vi "输入数据解析.vi"(0 "单个参数补充":dbl, 1 "从板号":dbl=1.0, 2 "主板二维码":string="BNET01", 3 "从板二维码":string="BNET01", 5 "主板引用":refnum<vi>, 7 "从板引用":refnum<vi>, 9 "主板选项":string="三级故障阀值", 11 "枚举":enum16{"主板", "从板"}(ring), 12 "快换":bool caption="快换写入") -> (4 "输出数组":dbl[][](array[numeric]), 6 "数组长度":dbl[](array[numeric]), 8 "循环次数":i32, 10 "命令":u32, 14 "名称":string[](array[string]), 15 "命令序号":u32[](array[numeric]))   [LabVIEW 2013] (continued)
          n4752 = Build Array(w12196) -> (w12195:dbl[][])
          n4753 = Build Array("二级故障阀值") -> (w12186:string[])
        }
        frame "SOC过低(3)" {
          n4754 = Unbundle By Name(w12405) -> ("一级故障 3"=w12406:refnum<vi>)
          n4755 = property class="Clust (严格)"(reference=w12406) -> ("Value"=w12404:T4)  [unwired: 1 in, 2 out]
          n4756 = for {
            N: 17 -> [_]
            tunnel: w12404 -> [w12416]
            shift-right: [w12413] -> w12410
            shift-left: dbl[] [] -> [w12414]
            i -> [w12417]
            n4757 = case shown="12" w12417 {
              tunnel: w12416 -> [w12418 w12429 w12440 w12450 w12460 w12470 w12482 w12494 w12506 w12518 w12530 w12542 w12554 w12566 w12573 w12582 w12591]
              tunnel: [w12419 w12430 w12441 w12451 w12461 w12472 w12484 w12496 w12508 w12520 w12532 w12543 w12556 w12568 w12572 w12581 w12593] -> w12415
              frame 0, Default {
                # "总电压过高"
                n4758 = disable-structure shown="启用" {
                  disable-tunnel: [w12425 w12428] -> w12421
                  disable-tunnel: [w12424 w12428] -> w12420
                  disable-tunnel: w12418 -> [w12423 _]
                  frame Disabled {
                    n4759 = Unbundle By Name(w12423) -> ("总电压过高"=w12422:dbl)
                    n4760 = call "输入分辨率计算-EV05.vi"("1字节?"=FALSE, "数值"=w12422, "分辨率"=0.1) -> ("低字节"=w12425:dbl, "高字节1"=w12424:dbl)  [unwired: 2 in, 5 out]
                  }
                  frame Enabled {
                    w12428 = 255 ("高字节1")
                  }
                }
                n4761 = Build Array(w12420, w12421) -> (w12419:i32[])
              }
              frame 1 {
                # "总电压过低"
                n4762 = disable-structure shown="启用" {
                  disable-tunnel: [w12436 w12439] -> w12432
                  disable-tunnel: [w12435 w12439] -> w12431
                  disable-tunnel: w12429 -> [w12434 _]
                  frame Disabled {
                    n4763 = Unbundle By Name(w12434) -> ("总电压过低"=w12433:dbl)
                    n4764 = call "输入分辨率计算-EV05.vi"("1字节?"=FALSE, "数值"=w12433, "分辨率"=0.1) -> ("低字节"=w12436:dbl, "高字节1"=w12435:dbl)  [unwired: 2 in, 5 out]
                  }
                  frame Enabled {
                    w12439 = 255 ("高字节1")
                  }
                }
                n4765 = Build Array(w12431, w12432) -> (w12430:i32[])
              }
              frame 2 {
                # "温度过高"
                n4766 = disable-structure shown="启用" {
                  disable-tunnel: [w12446 255 ("高字节1")] -> w12442
                  disable-tunnel: w12440 -> [w12444 _]
                  frame Disabled {
                    n4767 = Unbundle By Name(w12444) -> ("温度过高"=w12443:dbl)
                    n4768 = call "输入分辨率计算-EV05.vi"("1字节?"=TRUE, "数值"=w12443, "偏移量"=-40.0, "分辨率"=1.0) -> ("高字节1"=w12446:dbl)  [unwired: 1 in, 6 out]
                  }
                  frame Enabled {
                  }
                }
                n4769 = Build Array(w12442) -> (w12441:i32[])
              }
              frame 3 {
                # "温度过低"
                n4770 = disable-structure shown="启用" {
                  disable-tunnel: [w12456 255 ("高字节1")] -> w12452
                  disable-tunnel: w12450 -> [w12454 _]
                  frame Disabled {
                    n4771 = Unbundle By Name(w12454) -> ("温度过低"=w12453:dbl)
                    n4772 = call "输入分辨率计算-EV05.vi"("1字节?"=TRUE, "数值"=w12453, "偏移量"=-40.0, "分辨率"=1.0) -> ("高字节1"=w12456:dbl)  [unwired: 1 in, 6 out]
                  }
                  frame Enabled {
                  }
                }
                n4773 = Build Array(w12452) -> (w12451:i32[])
              }
              frame 4 {
                # "整组温度不均衡"
                n4774 = disable-structure shown="启用" {
                  disable-tunnel: [w12466 255 ("高字节1")] -> w12462
                  disable-tunnel: w12460 -> [w12464 _]
                  frame Disabled {
                    n4775 = Unbundle By Name(w12464) -> ("整组温度不均衡"=w12463:dbl)
                    n4776 = call "输入分辨率计算-EV05.vi"("1字节?"=TRUE, "数值"=w12463, "偏移量"=0.0, "分辨率"=1.0) -> ("高字节1"=w12466:dbl)  [unwired: 1 in, 6 out]
                  }
                  frame Enabled {
                  }
                }
                n4777 = Build Array(w12462) -> (w12461:i32[])
              }
              frame 5 {
                # "单组电压不均衡"
                n4778 = disable-structure shown="启用" {
                  disable-tunnel: [w12478 w12481] -> w12473
                  disable-tunnel: [w12476 w12481] -> w12471
                  disable-tunnel: w12470 -> [w12475 _]
                  frame Disabled {
                    n4779 = Unbundle By Name(w12475) -> ("单组电压不均衡"=w12474:dbl)
                    n4780 = call "输入分辨率计算-EV05.vi"("1字节?"=FALSE, "数值"=w12474, "偏移量"=0.0, "分辨率"=0.001) -> ("低字节"=w12476:dbl, "高字节1"=w12478:dbl)  [unwired: 1 in, 5 out]
                  }
                  frame Enabled {
                    w12481 = 255 ("高字节1")
                  }
                }
                n4781 = Build Array(w12473, w12471) -> (w12472:i32[])
              }
              frame 6 {
                # "整组电压不均衡"
                n4782 = disable-structure shown="启用" {
                  disable-tunnel: [w12490 w12493] -> w12485
                  disable-tunnel: [w12488 w12493] -> w12483
                  disable-tunnel: w12482 -> [w12487 _]
                  frame Disabled {
                    n4783 = Unbundle By Name(w12487) -> ("整组电压不均衡"=w12486:dbl)
                    n4784 = call "输入分辨率计算-EV05.vi"("1字节?"=FALSE, "数值"=w12486, "偏移量"=0.0, "分辨率"=0.001) -> ("低字节"=w12488:dbl, "高字节1"=w12490:dbl)  [unwired: 1 in, 5 out]
                  }
                  frame Enabled {
                    w12493 = 255 ("高字节1")
                  }
                }
                n4785 = Build Array(w12485, w12483) -> (w12484:i32[])
              }
              frame 7 {
                # "单体电压过高"
                n4786 = disable-structure shown="启用" {
                  disable-tunnel: [w12502 w12505] -> w12497
                  disable-tunnel: [w12500 w12505] -> w12495
                  disable-tunnel: w12494 -> [w12499 _]
                  frame Disabled {
                    n4787 = Unbundle By Name(w12499) -> ("单体电压过高"=w12498:dbl)
                    n4788 = call "输入分辨率计算-EV05.vi"("1字节?"=FALSE, "数值"=w12498, "偏移量"=0.0, "分辨率"=0.001) -> ("低字节"=w12500:dbl, "高字节1"=w12502:dbl)  [unwired: 1 in, 5 out]
                  }
                  frame Enabled {
                    w12505 = 255 ("高字节1")
                  }
                }
                n4789 = Build Array(w12497, w12495) -> (w12496:i32[])
              }
              frame 8 {
                # "单体电压过低"
                n4790 = disable-structure shown="启用" {
                  disable-tunnel: [w12514 w12517] -> w12509
                  disable-tunnel: [w12512 w12517] -> w12507
                  disable-tunnel: w12506 -> [w12511 _]
                  frame Disabled {
                    n4791 = Unbundle By Name(w12511) -> ("单体电压过低"=w12510:dbl)
                    n4792 = call "输入分辨率计算-EV05.vi"("1字节?"=FALSE, "数值"=w12510, "偏移量"=0.0, "分辨率"=0.001) -> ("低字节"=w12512:dbl, "高字节1"=w12514:dbl)  [unwired: 1 in, 5 out]
                  }
                  frame Enabled {
                    w12517 = 255 ("高字节1")
                  }
                }
                n4793 = Build Array(w12509, w12507) -> (w12508:i32[])
              }
              frame 9 {
                # "充电电流过高"
                n4794 = disable-structure shown="启用" {
                  disable-tunnel: [w12526 w12529] -> w12521
                  disable-tunnel: [w12524 w12529] -> w12519
                  disable-tunnel: w12518 -> [w12523 _]
                  frame Disabled {
                    n4795 = Unbundle By Name(w12523) -> ("充电电流过高"=w12522:dbl)
                    n4796 = call "输入分辨率计算-EV05.vi"("1字节?"=FALSE, "数值"=w12522, "偏移量"=-3000.0, "分辨率"=0.1) -> ("低字节"=w12524:dbl, "高字节1"=w12526:dbl)  [unwired: 1 in, 5 out]
                  }
                  frame Enabled {
                    w12529 = 255 ("高字节1")
                  }
                }
                n4797 = Build Array(w12521, w12519) -> (w12520:i32[])
              }
              frame 10 {
                # "放电电流过高"
                n4798 = disable-structure shown="启用" {
                  disable-tunnel: [w12538 w12541] -> w12533
                  disable-tunnel: [w12536 w12541] -> w12531
                  disable-tunnel: w12530 -> [w12535 _]
                  frame Disabled {
                    n4799 = Unbundle By Name(w12535) -> ("放电电流过高"=w12534:dbl)
                    n4800 = call "输入分辨率计算-EV05.vi"("1字节?"=FALSE, "数值"=w12534, "偏移量"=-3000.0, "分辨率"=0.1) -> ("低字节"=w12536:dbl, "高字节1"=w12538:dbl)  [unwired: 1 in, 5 out]
                  }
                  frame Enabled {
                    w12541 = 255 ("高字节1")
                  }
                }
                n4801 = Build Array(w12533, w12531) -> (w12532:i32[])
              }
              frame 11 {
                # "单组温度不均衡"
                n4802 = disable-structure shown="启用" {
                  disable-tunnel: [w12548 255 ("高字节1")] -> w12544
                  disable-tunnel: w12542 -> [w12546 _]
                  frame Disabled {
                    n4803 = Unbundle By Name(w12546) -> ("单组温度不均衡"=w12545:dbl)
                    n4804 = call "输入分辨率计算-EV05.vi"("1字节?"=TRUE, "数值"=w12545, "偏移量"=0.0, "分辨率"=1.0) -> ("高字节1"=w12548:dbl)  [unwired: 1 in, 6 out]
                  }
                  frame Enabled {
                  }
                }
                n4805 = Build Array(w12544) -> (w12543:i32[])
              }
              frame 12 {
                # "SOC过高"
                n4806 = Unbundle By Name(w12554) -> ("SOC过高"=w12553:dbl)
                n4807 = call "输入分辨率计算-EV05.vi"("1字节?"=FALSE, "数值"=w12553, "偏移量"=0.0, "分辨率"=0.1) -> ()  [unwired: 1 in, 7 out]
                n4808 = disable-structure shown="启用" {
                  disable-tunnel: _ -> [w12560 _]
                  disable-tunnel: [w12560 255 ("高字节1")] -> w12552
                  disable-tunnel: [w12559 i32[] [] ("低位子数组")] -> _
                  disable-tunnel: _ -> [w12559 _]
                  frame Disabled {
                  }
                  frame Enabled {
                  }
                }
                n4809 = Build Array(w12552, w12552) -> (w12556:i32[])
              }
              frame 13 {
                n4810 = Unbundle By Name(w12566) -> ("SOC过低"=w12565:dbl)
                n4811 = call "输入分辨率计算-EV05.vi"("1字节?"=FALSE, "数值"=w12565, "偏移量"=0.0, "分辨率"=0.1) -> ("低字节"=w12563:dbl, "高字节1"=w12564:dbl)  [unwired: 1 in, 5 out]
                n4812 = Build Array(w12564, w12563) -> (w12568:dbl[])
              }
              frame 14 {
                # "内阻过大"
                n4813 = disable-structure shown="启用" {
                  disable-tunnel: w12573 -> [w12578 _]
                  disable-tunnel: [w12574 255 ("高字节1")] -> w12571
                  frame Disabled {
                    n4814 = Unbundle By Name(w12578) -> ("内阻过大"=w12577:dbl)
                    n4815 = call "输入分辨率计算-EV05.vi"("1字节?"=TRUE, "数值"=w12577, "分辨率"=0.1) -> ("高字节1"=w12574:dbl)  [unwired: 2 in, 6 out]
                  }
                  frame Enabled {
                  }
                }
                n4816 = Build Array(w12571) -> (w12572:i32[])
              }
              frame 15 {
                # "极柱温度过高"
                n4817 = disable-structure shown="启用" {
                  disable-tunnel: w12582 -> [w12588 _]
                  disable-tunnel: [w12584 255 ("高字节1")] -> w12580
                  frame Disabled {
                    n4818 = Unbundle By Name(w12588) -> ("极柱温度过高"=w12587:dbl)
                    n4819 = call "输入分辨率计算-EV05.vi"("1字节?"=TRUE, "数值"=w12587, "偏移量"=-40.0, "分辨率"=1.0) -> ("高字节1"=w12584:dbl)  [unwired: 1 in, 6 out]
                  }
                  frame Enabled {
                  }
                }
                n4820 = Build Array(w12580) -> (w12581:i32[])
              }
              frame 16 {
                # "SOH过低"
                n4821 = disable-structure shown="启用" {
                  disable-tunnel: [w12605 w12613] -> w12592
                  disable-tunnel: w12591 -> [w12602 _]
                  disable-tunnel: [w12594 w12613] -> w12590
                  frame Disabled {
                    n4822 = Unbundle By Name(w12602) -> ("SOH过低"=w12601:dbl)
                    n4823 = call "输入分辨率计算-EV05.vi"("1字节?"=FALSE, "数值"=w12601, "偏移量"=0.0, "分辨率"=0.1) -> ("低字节"=w12603:dbl, "高字节1"=w12604:dbl)  [unwired: 1 in, 5 out]
                    n4824 = call "二进制解析-8.6.vi"("索引"=4, "数值"=w12604) -> ("低位子数组"=w12607:i32[])  [unwired: 3 out]
                    n4825 = call "二进制解析-8.6.vi"("索引"=4, "数值"=w12603) -> ("低位子数组"=w12596:i32[], "高位子数组"=w12606:i32[])  [unwired: 2 out]
                    n4826 = call "二进制解析-8.6.vi"("索引"=4, "数值"=0) -> ("低位子数组"=w12597:i32[])  [unwired: 3 out]
                    n4827 = Insert Into Array(array=w12607, new element=w12606) -> (w12600:i32[])  [unwired: 1 in]
                    n4828 = Insert Into Array(array=w12596, new element=w12597) -> (w12595:i32[])  [unwired: 1 in]
                    n4829 = call "数值二进制转十进制-8.6.vi"("子数组"=w12600) -> ("十进制数值"=w12605:i32)  [unwired: 4 out]
                    n4830 = call "数值二进制转十进制-8.6.vi"("子数组"=w12595) -> ("十进制数值"=w12594:i32)  [unwired: 4 out]
                  }
                  frame Enabled {
                    w12613 = 255 ("高字节1")
                  }
                }
                n4831 = Build Array(w12592, w12590) -> (w12593:i32[])
              }
            }
            n4832 = Insert Into Array(array=w12414, new element=w12415) -> (w12413:dbl[])  [unwired: 1 in]
          }
          n4833 = Build Array(w12410) -> (w12409:dbl[][])
          n4834 = Build Array("三级故障阀值") -> (w12400:string[])
        }
        frame "二级故障阀值" {
          n4835 = Unbundle By Name(w12619) -> ("一级故障 2"=w12620:refnum<vi>)
          n4836 = property class="Clust (严格)"(reference=w12620) -> ("Value"=w12618:T4)  [unwired: 1 in, 2 out]
          n4837 = for {
            N: 17 -> [_]
            tunnel: w12618 -> [w12630]
            shift-right: [w12627] -> w12624
            shift-left: dbl[] [] -> [w12628]
            i -> [w12631]
            n4838 = case shown="4" w12631 {
              tunnel: w12630 -> [w12633 w12640 w12647 w12654 w12661 w12667 w12675 w12683 w12691 w12699 w12707 w12715 w12723 w12731 w12741 w12748 w12752]
              tunnel: [w12634 w12641 w12649 w12656 w12662 w12670 w12678 w12686 w12694 w12702 w12710 w12716 w12725 w12733 w12740 w12747 w12754] -> w12629
              frame 0, Default {
                # "总电压过高"
                n4839 = Unbundle By Name(w12633) -> ("总电压过高"=w12632:dbl)
                n4840 = call "输入分辨率计算-EV05.vi"("1字节?"=FALSE, "数值"=w12632, "分辨率"=0.1) -> ("低字节"=w12636:dbl, "高字节1"=w12635:dbl)  [unwired: 2 in, 5 out]
                n4841 = Build Array(w12635, w12636) -> (w12634:dbl[])
              }
              frame 1 {
                # "总电压过低"
                n4842 = Unbundle By Name(w12640) -> ("总电压过低"=w12639:dbl)
                n4843 = call "输入分辨率计算-EV05.vi"("1字节?"=FALSE, "数值"=w12639, "分辨率"=0.1) -> ("低字节"=w12643:dbl, "高字节1"=w12642:dbl)  [unwired: 2 in, 5 out]
                n4844 = Build Array(w12642, w12643) -> (w12641:dbl[])
              }
              frame 2 {
                # "温度过高"
                n4845 = Unbundle By Name(w12647) -> ("温度过高"=w12646:dbl)
                n4846 = call "输入分辨率计算-EV05.vi"("1字节?"=TRUE, "数值"=w12646, "偏移量"=-40.0, "分辨率"=1.0) -> ("高字节1"=w12650:dbl)  [unwired: 1 in, 6 out]
                n4847 = Build Array(w12650) -> (w12649:dbl[])
              }
              frame 3 {
                # "温度过低"
                n4848 = Unbundle By Name(w12654) -> ("温度过低"=w12653:dbl)
                n4849 = call "输入分辨率计算-EV05.vi"("1字节?"=TRUE, "数值"=w12653, "偏移量"=-40.0, "分辨率"=1.0) -> ("高字节1"=w12657:dbl)  [unwired: 1 in, 6 out]
                n4850 = Build Array(w12657) -> (w12656:dbl[])
              }
              frame 4 {
                # "整组温度不均衡"
                n4851 = Unbundle By Name(w12661) -> ("整组温度不均衡"=w12660:dbl)
                n4852 = call "输入分辨率计算-EV05.vi"("1字节?"=TRUE, "数值"=w12660, "分辨率"=1.0) -> ("高字节1"=w12663:dbl)  [unwired: 2 in, 6 out]
                n4853 = Build Array(w12663) -> (w12662:dbl[])
              }
              frame 5 {
                # "单组电压不均衡"
                n4854 = Unbundle By Name(w12667) -> ("单组电压不均衡"=w12666:dbl)
                n4855 = call "输入分辨率计算-EV05.vi"("1字节?"=FALSE, "数值"=w12666, "偏移量"=0.0, "分辨率"=0.001) -> ("低字节"=w12668:dbl, "高字节1"=w12671:dbl)  [unwired: 1 in, 5 out]
                n4856 = Build Array(w12671, w12668) -> (w12670:dbl[])
              }
              frame 6 {
                # "整组电压不均衡"
                n4857 = Unbundle By Name(w12675) -> ("整组电压不均衡"=w12674:dbl)
                n4858 = call "输入分辨率计算-EV05.vi"("1字节?"=FALSE, "数值"=w12674, "偏移量"=0.0, "分辨率"=0.001) -> ("低字节"=w12676:dbl, "高字节1"=w12679:dbl)  [unwired: 1 in, 5 out]
                n4859 = Build Array(w12679, w12676) -> (w12678:dbl[])
              }
              frame 7 {
                # "单体电压过高"
                n4860 = Unbundle By Name(w12683) -> ("单体电压过高"=w12682:dbl)
                n4861 = call "输入分辨率计算-EV05.vi"("1字节?"=FALSE, "数值"=w12682, "偏移量"=0.0, "分辨率"=0.001) -> ("低字节"=w12684:dbl, "高字节1"=w12687:dbl)  [unwired: 1 in, 5 out]
                n4862 = Build Array(w12687, w12684) -> (w12686:dbl[])
              }
              frame 8 {
                # "单体电压过低"
                n4863 = Unbundle By Name(w12691) -> ("单体电压过低"=w12690:dbl)
                n4864 = call "输入分辨率计算-EV05.vi"("1字节?"=FALSE, "数值"=w12690, "偏移量"=0.0, "分辨率"=0.001) -> ("低字节"=w12692:dbl, "高字节1"=w12695:dbl)  [unwired: 1 in, 5 out]
                n4865 = Build Array(w12695, w12692) -> (w12694:dbl[])
              }
              frame 9 {
                # "充电电流过高"
                n4866 = Unbundle By Name(w12699) -> ("充电电流过高"=w12698:dbl)
                n4867 = call "输入分辨率计算-EV05.vi"("1字节?"=FALSE, "数值"=w12698, "偏移量"=0.0, "分辨率"=0.1) -> ("低字节"=w12700:dbl, "高字节1"=w12703:dbl)  [unwired: 1 in, 5 out]
                n4868 = Build Array(w12703, w12700) -> (w12702:dbl[])
              }
              frame 10 {
                # "放电电流过高"
                n4869 = Unbundle By Name(w12707) -> ("放电电流过高"=w12706:dbl)
                n4870 = call "输入分辨率计算-EV05.vi"("1字节?"=FALSE, "数值"=w12706, "偏移量"=0.0, "分辨率"=0.1) -> ("低字节"=w12708:dbl, "高字节1"=w12711:dbl)  [unwired: 1 in, 5 out]
                n4871 = Build Array(w12711, w12708) -> (w12710:dbl[])
              }
              frame 11 {
                # "单组温度不均衡"
                n4872 = Unbundle By Name(w12715) -> ("单组温度不均衡"=w12714:dbl)
                n4873 = call "输入分辨率计算-EV05.vi"("1字节?"=TRUE, "数值"=w12714, "分辨率"=1.0) -> ("高字节1"=w12717:dbl)  [unwired: 2 in, 6 out]
                n4874 = Build Array(w12717) -> (w12716:dbl[])
              }
              frame 12 {
                # "SOC过高"
                n4875 = Unbundle By Name(w12723) -> ("SOC过高"=w12722:dbl)
                n4876 = call "输入分辨率计算-EV05.vi"("1字节?"=FALSE, "数值"=w12722, "偏移量"=0.0, "分辨率"=0.1) -> ("低字节"=w12720:dbl, "高字节1"=w12721:dbl)  [unwired: 1 in, 5 out]
                n4877 = Build Array(w12721, w12720) -> (w12725:dbl[])
              }
              frame 13 {
                # "SOC过低"
                n4878 = Unbundle By Name(w12731) -> ("SOC过低"=w12730:dbl)
                n4879 = call "输入分辨率计算-EV05.vi"("1字节?"=FALSE, "数值"=w12730, "偏移量"=0.0, "分辨率"=0.1) -> ("低字节"=w12728:dbl, "高字节1"=w12729:dbl)  [unwired: 1 in, 5 out]
                n4880 = Build Array(w12729, w12728) -> (w12733:dbl[])
              }
              frame 14 {
                # "内阻过大"
                n4881 = Unbundle By Name(w12741) -> ("内阻过大"=w12739:dbl)
                n4882 = call "输入分辨率计算-EV05.vi"("1字节?"=TRUE, "数值"=w12739, "分辨率"=0.1) -> ("高字节1"=w12736:dbl)  [unwired: 2 in, 6 out]
                n4883 = Build Array(w12736) -> (w12740:dbl[])
              }
              frame 15 {
                # "极柱温度过高"
                n4884 = Unbundle By Name(w12748) -> ("极柱温度过高"=w12746:dbl)
                n4885 = call "输入分辨率计算-EV05.vi"("1字节?"=TRUE, "数值"=w12746, "偏移量"=-40.0, "分辨率"=1.0) -> ("高字节1"=w12743:dbl)  [unwired: 1 in, 6 out]
                n4886 = Build Array(w12743) -> (w12747:dbl[])
              }
              frame 16 {
                # "SOH过低"
                n4887 = Unbundle By Name(w12752) -> ("SOH过低"=w12751:dbl)
                n4888 = call "输入分辨率计算-EV05.vi"("1字节?"=FALSE, "数值"=w12751, "偏移量"=0.0, "分辨率"=0.1) -> ("低字节"=w12749:dbl, "高字节1"=w12750:dbl)  [unwired: 1 in, 5 out]
                n4889 = Build Array(w12750, w12749) -> (w12754:dbl[])
              }
            }
            n4890 = Insert Into Array(array=w12628, new element=w12629) -> (w12627:dbl[])  [unwired: 1 in]
          }
          n4891 = Build Array(w12624) -> (w12623:dbl[][])
          n4892 = Build Array("二级故障阀值") -> (w12614:string[])
        }
        frame "三级故障阀值" {
          n4893 = Unbundle By Name(w12762) -> ("一级故障 3"=w12763:refnum<vi>)
          n4894 = property class="Clust (严格)"(reference=w12763) -> ("Value"=w12761:T4)  [unwired: 1 in, 2 out]
          n4895 = for {
            N: 17 -> [_]
            tunnel: w12761 -> [w12773]
            shift-right: [w12770] -> w12767
            shift-left: dbl[] [] -> [w12771]
            i -> [w12774]
            n4896 = case shown="11" w12774 {
              tunnel: w12773 -> [w12776 w12783 w12790 w12797 w12804 w12810 w12818 w12826 w12834 w12842 w12850 w12858 w12866 w12874 w12884 w12891 w12895]
              tunnel: [w12777 w12784 w12792 w12799 w12805 w12813 w12821 w12829 w12837 w12845 w12853 w12859 w12868 w12876 w12883 w12890 w12897] -> w12772
              frame 0, Default {
                # "总电压过高"
                n4897 = Unbundle By Name(w12776) -> ("总电压过高"=w12775:dbl)
                n4898 = call "输入分辨率计算-EV05.vi"("1字节?"=FALSE, "数值"=w12775, "分辨率"=0.1) -> ("低字节"=w12779:dbl, "高字节1"=w12778:dbl)  [unwired: 2 in, 5 out]
                n4899 = Build Array(w12778, w12779) -> (w12777:dbl[])
              }
              frame 1 {
                # "总电压过低"
                n4900 = Unbundle By Name(w12783) -> ("总电压过低"=w12782:dbl)
                n4901 = call "输入分辨率计算-EV05.vi"("1字节?"=FALSE, "数值"=w12782, "分辨率"=0.1) -> ("低字节"=w12786:dbl, "高字节1"=w12785:dbl)  [unwired: 2 in, 5 out]
                n4902 = Build Array(w12785, w12786) -> (w12784:dbl[])
              }
              frame 2 {
                # "温度过高"
                n4903 = Unbundle By Name(w12790) -> ("温度过高"=w12789:dbl)
                n4904 = call "输入分辨率计算-EV05.vi"("1字节?"=TRUE, "数值"=w12789, "偏移量"=-40.0, "分辨率"=1.0) -> ("高字节1"=w12793:dbl)  [unwired: 1 in, 6 out]
                n4905 = Build Array(w12793) -> (w12792:dbl[])
              }
              frame 3 {
                # "温度过低"
                n4906 = Unbundle By Name(w12797) -> ("温度过低"=w12796:dbl)
                n4907 = call "输入分辨率计算-EV05.vi"("1字节?"=TRUE, "数值"=w12796, "偏移量"=-40.0, "分辨率"=1.0) -> ("高字节1"=w12800:dbl)  [unwired: 1 in, 6 out]
                n4908 = Build Array(w12800) -> (w12799:dbl[])
              }
              frame 4 {
                # "整组温度不均衡"
                n4909 = Unbundle By Name(w12804) -> ("整组温度不均衡"=w12803:dbl)
                n4910 = call "输入分辨率计算-EV05.vi"("1字节?"=TRUE, "数值"=w12803, "分辨率"=1.0) -> ("高字节1"=w12806:dbl)  [unwired: 2 in, 6 out]
                n4911 = Build Array(w12806) -> (w12805:dbl[])
              }
              frame 5 {
                # "单组电压不均衡"
                n4912 = Unbundle By Name(w12810) -> ("单组电压不均衡"=w12809:dbl)
                n4913 = call "输入分辨率计算-EV05.vi"("1字节?"=FALSE, "数值"=w12809, "偏移量"=0.0, "分辨率"=0.001) -> ("低字节"=w12811:dbl, "高字节1"=w12814:dbl)  [unwired: 1 in, 5 out]
                n4914 = Build Array(w12814, w12811) -> (w12813:dbl[])
              }
              frame 6 {
                # "整组电压不均衡"
                n4915 = Unbundle By Name(w12818) -> ("整组电压不均衡"=w12817:dbl)
                n4916 = call "输入分辨率计算-EV05.vi"("1字节?"=FALSE, "数值"=w12817, "偏移量"=0.0, "分辨率"=0.001) -> ("低字节"=w12819:dbl, "高字节1"=w12822:dbl)  [unwired: 1 in, 5 out]
                n4917 = Build Array(w12822, w12819) -> (w12821:dbl[])
              }
              frame 7 {
                # "单体电压过高"
                n4918 = Unbundle By Name(w12826) -> ("单体电压过高"=w12825:dbl)
                n4919 = call "输入分辨率计算-EV05.vi"("1字节?"=FALSE, "数值"=w12825, "偏移量"=0.0, "分辨率"=0.001) -> ("低字节"=w12827:dbl, "高字节1"=w12830:dbl)  [unwired: 1 in, 5 out]
                n4920 = Build Array(w12830, w12827) -> (w12829:dbl[])
              }
              frame 8 {
                # "单体电压过低"
                n4921 = Unbundle By Name(w12834) -> ("单体电压过低"=w12833:dbl)
                n4922 = call "输入分辨率计算-EV05.vi"("1字节?"=FALSE, "数值"=w12833, "偏移量"=0.0, "分辨率"=0.001) -> ("低字节"=w12835:dbl, "高字节1"=w12838:dbl)  [unwired: 1 in, 5 out]
                n4923 = Build Array(w12838, w12835) -> (w12837:dbl[])
              }
              frame 9 {
                # "充电电流过高"
                n4924 = Unbundle By Name(w12842) -> ("充电电流过高"=w12841:dbl)
                n4925 = call "输入分辨率计算-EV05.vi"("1字节?"=FALSE, "数值"=w12841, "偏移量"=0.0, "分辨率"=0.1) -> ("低字节"=w12843:dbl, "高字节1"=w12846:dbl)  [unwired: 1 in, 5 out]
                n4926 = Build Array(w12846, w12843) -> (w12845:dbl[])
              }
              frame 10 {
                # "放电电流过高"
                n4927 = Unbundle By Name(w12850) -> ("放电电流过高"=w12849:dbl)
                n4928 = call "输入分辨率计算-EV05.vi"("1字节?"=FALSE, "数值"=w12849, "偏移量"=0.0, "分辨率"=0.1) -> ("低字节"=w12851:dbl, "高字节1"=w12854:dbl)  [unwired: 1 in, 5 out]
                n4929 = Build Array(w12854, w12851) -> (w12853:dbl[])
              }
              frame 11 {
                # "单组温度不均衡"
                n4930 = Unbundle By Name(w12858) -> ("单组温度不均衡"=w12857:dbl)
                n4931 = call "输入分辨率计算-EV05.vi"("1字节?"=TRUE, "数值"=w12857, "分辨率"=1.0) -> ("高字节1"=w12860:dbl)  [unwired: 2 in, 6 out]
                n4932 = Build Array(w12860) -> (w12859:dbl[])
              }
              frame 12 {
                # "SOC过高"
                n4933 = Unbundle By Name(w12866) -> ("SOC过高"=w12865:dbl)
                n4934 = call "输入分辨率计算-EV05.vi"("1字节?"=FALSE, "数值"=w12865, "偏移量"=0.0, "分辨率"=0.1) -> ("低字节"=w12863:dbl, "高字节1"=w12864:dbl)  [unwired: 1 in, 5 out]
                n4935 = Build Array(w12864, w12863) -> (w12868:dbl[])
              }
              frame 13 {
                # "SOC过低"
                n4936 = Unbundle By Name(w12874) -> ("SOC过低"=w12873:dbl)
                n4937 = call "输入分辨率计算-EV05.vi"("1字节?"=FALSE, "数值"=w12873, "偏移量"=0.0, "分辨率"=0.1) -> ("低字节"=w12871:dbl, "高字节1"=w12872:dbl)  [unwired: 1 in, 5 out]
                n4938 = Build Array(w12872, w12871) -> (w12876:dbl[])
              }
              frame 14 {
                # "内阻过大"
                n4939 = Unbundle By Name(w12884) -> ("内阻过大"=w12882:dbl)
                n4940 = call "输入分辨率计算-EV05.vi"("1字节?"=TRUE, "数值"=w12882, "分辨率"=0.1) -> ("高字节1"=w12879:dbl)  [unwired: 2 in, 6 out]
                n4941 = Build Array(w12879) -> (w12883:dbl[])
              }
              frame 15 {
                # "极柱温度过高"
                n4942 = Unbundle By Name(w12891) -> ("极柱温度过高"=w12889:dbl)
                n4943 = call "输入分辨率计算-EV05.vi"("1字节?"=TRUE, "数值"=w12889, "偏移量"=-40.0, "分辨率"=1.0) -> ("高字节1"=w12886:dbl)  [unwired: 1 in, 6 out]
                n4944 = Build Array(w12886) -> (w12890:dbl[])
              }
              frame 16 {
                # "SOH过低"
                n4945 = Unbundle By Name(w12895) -> ("SOH过低"=w12894:dbl)
                n4946 = call "输入分辨率计算-EV05.vi"("1字节?"=FALSE, "数值"=w12894, "偏移量"=0.0, "分辨率"=0.1) -> ("低字节"=w12892:dbl, "高字节1"=w12893:dbl)  [unwired: 1 in, 5 out]
                n4947 = Build Array(w12893, w12892) -> (w12897:dbl[])
              }
            }
            n4948 = Insert Into Array(array=w12771, new element=w12772) -> (w12770:dbl[])  [unwired: 1 in]
          }
          n4949 = Build Array(w12767) -> (w12766:dbl[][])
          n4950 = Build Array("三级故障阀值") -> (w12757:string[])
        }
        frame "加热控制参数" {
          n4951 = Unbundle By Name(w12921) -> ("加热控制参数"=w12922:refnum<vi>)
          n4952 = property class="Clust (严格)"(reference=w12922) -> ("Value"=w12920:T5)  [unwired: 1 in, 2 out]
          n4953 = Unbundle(w12920) -> ("风机开启温度"=w12915:dbl, "风机关闭温度"=w12914:dbl, "加热开启温度"=w12911:dbl, "加热关闭温度"=w12910:dbl, "风机开启温差"=w12904:dbl, "风机关闭温差"=w12903:dbl, "加热关闭温差"=w12900:dbl)
          n4954 = call "输入分辨率计算-EV05.vi"("1字节?"=TRUE, "数值 2"=w12910, "数值"=w12911, "偏移量"=-40.0, "分辨率"=1.0) -> ("高字节 2"=w12901:dbl, "高字节1"=w12902:dbl)  [unwired: 5 out]
          n4955 = call "输入分辨率计算-EV05.vi"("1字节?"=TRUE, "数值 2"=w12914, "数值"=w12915, "偏移量"=-40.0, "分辨率"=1.0) -> ("高字节 2"=w12908:dbl, "高字节1"=w12909:dbl)  [unwired: 5 out]
          n4956 = Build Array(w12909, w12908, w12904, w12903, w12902, w12901, w12900) -> (w12907:dbl[])
          n4957 = Build Array(w12907) -> (w12925:dbl[][])
        }
        frame "风机开启温度" {
          w12927 = 255 ("高字节1")
          n4958 = Unbundle By Name(w12943) -> ("加热控制参数"=w12944:refnum<vi>)
          n4959 = property class="Clust (严格)"(reference=w12944) -> ("Value"=w12942:T5)  [unwired: 1 in, 2 out]
          n4960 = Unbundle(w12942) -> ("风机开启温度"=w12937:dbl, "风机关闭温度"=w12936:dbl, "加热开启温度"=w12933:dbl, "加热关闭温度"=w12932:dbl)  [unwired: 3 out]
          n4961 = call "输入分辨率计算-EV05.vi"("1字节?"=TRUE, "数值 2"=w12932, "数值"=w12933, "偏移量"=-40.0, "分辨率"=1.0) -> ()  [unwired: 7 out]
          n4962 = call "输入分辨率计算-EV05.vi"("1字节?"=TRUE, "数值 2"=w12936, "数值"=w12937, "偏移量"=-40.0, "分辨率"=1.0) -> ("高字节1"=w12931:dbl)  [unwired: 6 out]
          n4963 = Build Array(w12931, w12927, w12927, w12927, w12927, w12927, w12927) -> (w12930:dbl[])
          n4964 = Build Array(w12930) -> (w12947:dbl[][])
        }
        frame "风机关闭温度" {
          w12949 = 255 ("高字节1")
          n4965 = Unbundle By Name(w12965) -> ("加热控制参数"=w12966:refnum<vi>)
          n4966 = property class="Clust (严格)"(reference=w12966) -> ("Value"=w12964:T5)  [unwired: 1 in, 2 out]
          n4967 = Unbundle(w12964) -> ("风机开启温度"=w12959:dbl, "风机关闭温度"=w12958:dbl, "加热开启温度"=w12955:dbl, "加热关闭温度"=w12954:dbl)  [unwired: 3 out]
          n4968 = call "输入分辨率计算-EV05.vi"("1字节?"=TRUE, "数值 2"=w12954, "数值"=w12955, "偏移量"=-40.0, "分辨率"=1.0) -> ()  [unwired: 7 out]
          n4969 = call "输入分辨率计算-EV05.vi"("1字节?"=TRUE, "数值 2"=w12958, "数值"=w12959, "偏移量"=-40.0, "分辨率"=1.0) -> ("高字节 2"=w12952:dbl)  [unwired: 6 out]
          n4970 = Build Array(w12949, w12952, w12949, w12949, w12949, w12949, w12949) -> (w12953:dbl[])
          n4971 = Build Array(w12953) -> (w12969:dbl[][])
        }
        frame "加热开启温度" {
          w12971 = 255 ("高字节1")
          n4972 = Unbundle By Name(w12987) -> ("加热控制参数"=w12988:refnum<vi>)
          n4973 = property class="Clust (严格)"(reference=w12988) -> ("Value"=w12986:T5)  [unwired: 1 in, 2 out]
          n4974 = Unbundle(w12986) -> ("风机开启温度"=w12981:dbl, "风机关闭温度"=w12980:dbl, "加热开启温度"=w12977:dbl, "加热关闭温度"=w12976:dbl)  [unwired: 3 out]
          n4975 = call "输入分辨率计算-EV05.vi"("1字节?"=TRUE, "数值 2"=w12976, "数值"=w12977, "偏移量"=-40.0, "分辨率"=1.0) -> ("高字节1"=w12972:dbl)  [unwired: 6 out]
          n4976 = call "输入分辨率计算-EV05.vi"("1字节?"=TRUE, "数值 2"=w12980, "数值"=w12981, "偏移量"=-40.0, "分辨率"=1.0) -> ()  [unwired: 7 out]
          n4977 = Build Array(w12971, w12971, w12971, w12971, w12972, w12971, w12971) -> (w12975:dbl[])
          n4978 = Build Array(w12975) -> (w12991:dbl[][])
        }
        frame "加热关闭温度" {
          w12993 = 255 ("高字节1")
          n4979 = Unbundle By Name(w13009) -> ("加热控制参数"=w13010:refnum<vi>)
          n4980 = property class="Clust (严格)"(reference=w13010) -> ("Value"=w13008:T5)  [unwired: 1 in, 2 out]
          n4981 = Unbundle(w13008) -> ("风机开启温度"=w13003:dbl, "风机关闭温度"=w13002:dbl, "加热开启温度"=w12999:dbl, "加热关闭温度"=w12998:dbl)  [unwired: 3 out]
          n4982 = call "输入分辨率计算-EV05.vi"("1字节?"=TRUE, "数值 2"=w12998, "数值"=w12999, "偏移量"=-40.0, "分辨率"=1.0) -> ("高字节 2"=w12994:dbl)  [unwired: 6 out]
          n4983 = call "输入分辨率计算-EV05.vi"("1字节?"=TRUE, "数值 2"=w13002, "数值"=w13003, "偏移量"=-40.0, "分辨率"=1.0) -> ()  [unwired: 7 out]
          n4984 = Build Array(w12993, w12993, w12993, w12993, w12993, w12994, w12993) -> (w12997:dbl[])
          n4985 = Build Array(w12997) -> (w13013:dbl[][])
        }
        frame "风机开启温差" {
          w13015 = 255 ("高字节1")
          n4986 = Unbundle By Name(w13031) -> ("加热控制参数"=w13032:refnum<vi>)
          n4987 = property class="Clust (严格)"(reference=w13032) -> ("Value"=w13030:T5)  [unwired: 1 in, 2 out]
          n4988 = Unbundle(w13030) -> ("风机开启温度"=w13025:dbl, "风机关闭温度"=w13024:dbl, "加热开启温度"=w13021:dbl, "加热关闭温度"=w13020:dbl, "风机开启温差"=w13016:dbl)  [unwired: 2 out]
          n4989 = call "输入分辨率计算-EV05.vi"("1字节?"=TRUE, "数值 2"=w13020, "数值"=w13021, "偏移量"=-40.0, "分辨率"=1.0) -> ()  [unwired: 7 out]
          n4990 = call "输入分辨率计算-EV05.vi"("1字节?"=TRUE, "数值 2"=w13024, "数值"=w13025, "偏移量"=-40.0, "分辨率"=1.0) -> ()  [unwired: 7 out]
          n4991 = Build Array(w13015, w13015, w13016, w13015, w13015, w13015, w13015) -> (w13019:dbl[])
          n4992 = Build Array(w13019) -> (w13035:dbl[][])
        }
        frame "风机关闭温差" {
          w13037 = 255 ("高字节1")
          n4993 = Unbundle By Name(w13053) -> ("加热控制参数"=w13054:refnum<vi>)
          n4994 = property class="Clust (严格)"(reference=w13054) -> ("Value"=w13052:T5)  [unwired: 1 in, 2 out]
          n4995 = Unbundle(w13052) -> ("风机开启温度"=w13047:dbl, "风机关闭温度"=w13046:dbl, "加热开启温度"=w13043:dbl, "加热关闭温度"=w13042:dbl, "风机关闭温差"=w13038:dbl)  [unwired: 2 out]
          n4996 = call "输入分辨率计算-EV05.vi"("1字节?"=TRUE, "数值 2"=w13042, "数值"=w13043, "偏移量"=-40.0, "分辨率"=1.0) -> ()  [unwired: 7 out]
          n4997 = call "输入分辨率计算-EV05.vi"("1字节?"=TRUE, "数值 2"=w13046, "数值"=w13047, "偏移量"=-40.0, "分辨率"=1.0) -> ()  [unwired: 7 out]
          n4998 = Build Array(w13037, w13037, w13037, w13038, w13037, w13037, w13037) -> (w13041:dbl[])
          n4999 = Build Array(w13041) -> (w13057:dbl[][])
        }
        frame "加热关闭温差" {
          w13060 = 255 ("高字节1")
          n5000 = Unbundle By Name(w13075) -> ("加热控制参数"=w13076:refnum<vi>)
          n5001 = property class="Clust (严格)"(reference=w13076) -> ("Value"=w13074:T5)  [unwired: 1 in, 2 out]
          n5002 = Unbundle(w13074) -> ("风机开启温度"=w13069:dbl, "风机关闭温度"=w13068:dbl, "加热开启温度"=w13065:dbl, "加热关闭温度"=w13064:dbl, "加热关闭温差"=w13059:dbl)  [unwired: 2 out]
          n5003 = call "输入分辨率计算-EV05.vi"("1字节?"=TRUE, "数值 2"=w13064, "数值"=w13065, "偏移量"=-40.0, "分辨率"=1.0) -> ()  [unwired: 7 out]
          n5004 = call "输入分辨率计算-EV05.vi"("1字节?"=TRUE, "数值 2"=w13068, "数值"=w13069, "偏移量"=-40.0, "分辨率"=1.0) -> ()  [unwired: 7 out]
          n5005 = Build Array(w13060, w13060, w13060, w13060, w13060, w13060, w13059) -> (w13063:dbl[])
          n5006 = Build Array(w13063) -> (w13079:dbl[][])
        }
        frame "充电控制参数" {
          n5007 = Unbundle By Name(w13084) -> ("充电控制参数"=w13085:refnum<vi>)
          n5008 = property class="Clust (严格)"(reference=w13085) -> ("Value"=w13083:T6)  [unwired: 1 in, 2 out]
          n5009 = for {
            N: 8 -> [_]
            tunnel: w13083 -> [w13095]
            shift-right: [w13097] -> w13089
            shift-left: dbl[] [] -> [w13093]
            i -> [w13096]
            n5010 = case shown="5" w13096 {
              tunnel: w13095 -> [w13099 w13106 w13113 w13121 w13128 w13135 w13143 w13150]
              tunnel: [w13100 w13107 w13115 w13123 w13130 w13138 w13145 w13152] -> w13094
              frame 0, Default {
                # "最大允许单体电压"
                n5011 = Unbundle By Name(w13099) -> ("最大允许单体电压"=w13098:dbl)
                n5012 = call "输入分辨率计算-EV05.vi"("1字节?"=FALSE, "数值"=w13098, "分辨率"=0.001) -> ("低字节"=w13101:dbl, "高字节1"=w13102:dbl)  [unwired: 2 in, 5 out]
                n5013 = Build Array(w13102, w13101) -> (w13100:dbl[])
              }
              frame 1 {
                # "最大允许总电压"
                n5014 = Unbundle By Name(w13106) -> ("最大允许总电压"=w13105:dbl)
                n5015 = call "输入分辨率计算-EV05.vi"("1字节?"=FALSE, "数值"=w13105, "分辨率"=0.1) -> ("低字节"=w13108:dbl, "高字节1"=w13109:dbl)  [unwired: 2 in, 5 out]
                n5016 = Build Array(w13109, w13108) -> (w13107:dbl[])
              }
              frame 2 {
                # "最大允许充电电流"
                n5017 = Unbundle By Name(w13113) -> ("最大允许充电电流"=w13112:dbl)
                n5018 = call "输入分辨率计算-EV05.vi"("1字节?"=FALSE, "数值"=w13112, "偏移量"=0.0, "分辨率"=0.1) -> ("低字节"=w13116:dbl, "高字节1"=w13117:dbl)  [unwired: 1 in, 5 out]
                n5019 = Build Array(w13117, w13116) -> (w13115:dbl[])
              }
              frame 3 {
                # "最小允许充电温度"
                n5020 = Unbundle By Name(w13121) -> ("最小允许充电温度"=w13120:dbl)
                n5021 = call "输入分辨率计算-EV05.vi"("1字节?"=TRUE, "数值"=w13120, "偏移量"=-40.0, "分辨率"=1.0) -> ("高字节1"=w13124:dbl)  [unwired: 1 in, 6 out]
                n5022 = Build Array(w13124) -> (w13123:dbl[])
              }
              frame 4 {
                # "最小充电电流"
                n5023 = Unbundle By Name(w13128) -> ("最小允许充电电流"=w13127:dbl)
                n5024 = call "输入分辨率计算-EV05.vi"("1字节?"=FALSE, "数值"=w13127, "分辨率"=0.1) -> ("低字节"=w13129:dbl, "高字节1"=w13131:dbl)  [unwired: 2 in, 5 out]
                n5025 = Build Array(w13131, w13129) -> (w13130:dbl[])
              }
              frame 5 {
                # "电流步长"
                n5026 = Unbundle By Name(w13135) -> ("电流步长"=w13134:dbl)
                n5027 = call "输入分辨率计算-EV05.vi"("1字节?"=FALSE, "数值"=w13134, "偏移量"=0.0, "分辨率"=0.1) -> ("低字节"=w13136:dbl, "高字节1"=w13139:dbl)  [unwired: 1 in, 5 out]
                n5028 = Build Array(w13139, w13136) -> (w13138:dbl[])
              }
              frame 6 {
                # "最小允许单体电压"
                n5029 = Unbundle By Name(w13143) -> ("最小允许单体电压"=w13142:dbl)
                n5030 = call "输入分辨率计算-EV05.vi"("1字节?"=FALSE, "数值"=w13142, "分辨率"=0.001) -> ("低字节"=w13144:dbl, "高字节1"=w13146:dbl)  [unwired: 2 in, 5 out]
                n5031 = Build Array(w13146, w13144) -> (w13145:dbl[])
              }
              frame 7 {
                # "最大允许充电温度"
                n5032 = Unbundle By Name(w13150) -> ("最大允许充电温度"=w13149:dbl)
                n5033 = call "输入分辨率计算-EV05.vi"("1字节?"=TRUE, "数值"=w13149, "偏移量"=-40.0, "分辨率"=1.0) -> ("高字节1"=w13153:dbl)  [unwired: 1 in, 6 out]
                n5034 = Build Array(w13153) -> (w13152:dbl[])
              }
            }
            n5035 = Insert Into Array(array=w13093, new element=w13094) -> (w13097:dbl[])  [unwired: 1 in]
          }
          n5036 = Build Array(w13089) -> (w13091:dbl[][])
        }
        frame "最大允许单体电压" {
          n5037 = Unbundle By Name(w13159) -> ("充电控制参数"=w13160:refnum<vi>)
          n5038 = property class="Clust (严格)"(reference=w13160) -> ("Value"=w13158:T6)  [unwired: 1 in, 2 out]
          n5039 = for {
            N: 8 -> [_]
            tunnel: w13158 -> [w13170]
            shift-right: [w13172] -> w13164
            shift-left: dbl[] [] -> [w13168]
            i -> [w13171]
            n5040 = case shown="0, 默认" w13171 {
              tunnel: w13170 -> [w13173 w13184 w13195 w13207 w13217 w13228 w13240 w13251]
              tunnel: [w13174 w13185 w13196 w13208 w13219 w13230 w13242 w13252] -> w13169
              frame 0, Default {
                # "最大允许单体电压"
                n5041 = disable-structure shown="启用" {
                  disable-tunnel: [w13180 w13183] -> w13176
                  disable-tunnel: [w13179 w13183] -> w13175
                  disable-tunnel: w13173 -> [w13178 _]
                  frame Enabled {
                    n5042 = Unbundle By Name(w13178) -> ("最大允许单体电压"=w13177:dbl)
                    n5043 = call "输入分辨率计算-EV05.vi"("1字节?"=FALSE, "数值"=w13177, "分辨率"=0.001) -> ("低字节"=w13179:dbl, "高字节1"=w13180:dbl)  [unwired: 2 in, 5 out]
                  }
                  frame Disabled {
                    w13183 = 255 ("高字节1")
                  }
                }
                n5044 = Build Array(w13176, w13175) -> (w13174:dbl[])
              }
              frame 1 {
                # "最大允许总电压"
                n5045 = disable-structure shown="启用" {
                  disable-tunnel: [w13191 w13194] -> w13187
                  disable-tunnel: [w13190 w13194] -> w13186
                  disable-tunnel: w13184 -> [w13189 _]
                  frame Disabled {
                    n5046 = Unbundle By Name(w13189) -> ("最大允许总电压"=w13188:dbl)
                    n5047 = call "输入分辨率计算-EV05.vi"("1字节?"=FALSE, "数值"=w13188, "分辨率"=0.1) -> ("低字节"=w13190:dbl, "高字节1"=w13191:dbl)  [unwired: 2 in, 5 out]
                  }
                  frame Enabled {
                    w13194 = 255 ("高字节1")
                  }
                }
                n5048 = Build Array(w13187, w13186) -> (w13185:i32[])
              }
              frame 2 {
                # "最大允许充电电流"
                n5049 = disable-structure shown="启用" {
                  disable-tunnel: [w13203 w13206] -> w13198
                  disable-tunnel: [w13202 w13206] -> w13197
                  disable-tunnel: w13195 -> [w13200 _]
                  frame Disabled {
                    n5050 = Unbundle By Name(w13200) -> ("最大允许充电电流"=w13199:dbl)
                    n5051 = call "输入分辨率计算-EV05.vi"("1字节?"=FALSE, "数值"=w13199, "偏移量"=-3000.0, "分辨率"=0.1) -> ("低字节"=w13202:dbl, "高字节1"=w13203:dbl)  [unwired: 1 in, 5 out]
                  }
                  frame Enabled {
                    w13206 = 255 ("高字节1")
                  }
                }
                n5052 = Build Array(w13198, w13197) -> (w13196:i32[])
              }
              frame 3 {
                # "最小允许充电温度"
                n5053 = disable-structure shown="启用" {
                  disable-tunnel: [w13213 255 ("高字节1")] -> w13209
                  disable-tunnel: w13207 -> [w13211 _]
                  frame Disabled {
                    n5054 = Unbundle By Name(w13211) -> ("最小允许温度"=w13210:dbl)
                    n5055 = call "输入分辨率计算-EV05.vi"("1字节?"=TRUE, "数值"=w13210, "偏移量"=-40.0, "分辨率"=1.0) -> ("高字节1"=w13213:dbl)  [unwired: 1 in, 6 out]
                  }
                  frame Enabled {
                  }
                }
                n5056 = Build Array(w13209) -> (w13208:i32[])
              }
              frame 4 {
                # "最小充电电流"
                n5057 = disable-structure shown="启用" {
                  disable-tunnel: [w13224 w13227] -> w13220
                  disable-tunnel: [w13223 w13227] -> w13218
                  disable-tunnel: w13217 -> [w13222 _]
                  frame Disabled {
                    n5058 = Unbundle By Name(w13222) -> ("最小充电电流"=w13221:dbl)
                    n5059 = call "输入分辨率计算-EV05.vi"("1字节?"=FALSE, "数值"=w13221, "分辨率"=0.1) -> ("低字节"=w13223:dbl, "高字节1"=w13224:dbl)  [unwired: 2 in, 5 out]
                  }
                  frame Enabled {
                    w13227 = 255 ("高字节1")
                  }
                }
                n5060 = Build Array(w13220, w13218) -> (w13219:i32[])
              }
              frame 5 {
                # "电流步长"
                n5061 = disable-structure shown="启用" {
                  disable-tunnel: [w13236 w13239] -> w13231
                  disable-tunnel: [w13234 w13239] -> w13229
                  disable-tunnel: w13228 -> [w13233 _]
                  frame Disabled {
                    n5062 = Unbundle By Name(w13233) -> ("电流步长"=w13232:dbl)
                    n5063 = call "输入分辨率计算-EV05.vi"("1字节?"=FALSE, "数值"=w13232, "偏移量"=0.0, "分辨率"=1.0) -> ("低字节"=w13234:dbl, "高字节1"=w13236:dbl)  [unwired: 1 in, 5 out]
                  }
                  frame Enabled {
                    w13239 = 255 ("高字节1")
                  }
                }
                n5064 = Build Array(w13231, w13229) -> (w13230:i32[])
              }
              frame 6 {
                # "最小允许单体电压"
                n5065 = disable-structure shown="启用" {
                  disable-tunnel: [w13247 w13250] -> w13243
                  disable-tunnel: [w13246 w13250] -> w13241
                  disable-tunnel: w13240 -> [w13245 _]
                  frame Disabled {
                    n5066 = Unbundle By Name(w13245) -> ("最小允许单体电压"=w13244:dbl)
                    n5067 = call "输入分辨率计算-EV05.vi"("1字节?"=FALSE, "数值"=w13244, "分辨率"=0.001) -> ("低字节"=w13246:dbl, "高字节1"=w13247:dbl)  [unwired: 2 in, 5 out]
                  }
                  frame Enabled {
                    w13250 = 255 ("高字节1")
                  }
                }
                n5068 = Build Array(w13243, w13241) -> (w13242:i32[])
              }
              frame 7 {
                # "最大允许充电温度"
                n5069 = disable-structure shown="启用" {
                  disable-tunnel: [w13257 255 ("高字节1")] -> w13253
                  disable-tunnel: w13251 -> [w13255 _]
                  frame Disabled {
                    n5070 = Unbundle By Name(w13255) -> ("最大允许充电温度"=w13254:dbl)
                    n5071 = call "输入分辨率计算-EV05.vi"("1字节?"=TRUE, "数值"=w13254, "偏移量"=-40.0, "分辨率"=1.0) -> ("高字节1"=w13257:dbl)  [unwired: 1 in, 6 out]
                  }
                  frame Enabled {
                  }
                }
                n5072 = Build Array(w13253) -> (w13252:i32[])
              }
            }
            n5073 = Insert Into Array(array=w13168, new element=w13169) -> (w13172:dbl[])  [unwired: 1 in]
          }
          n5074 = Build Array(w13164) -> (w13166:dbl[][])
        }
        frame "最大允许总电压" {
          n5075 = Unbundle By Name(w13264) -> ("充电控制参数"=w13265:refnum<vi>)
          n5076 = property class="Clust (严格)"(reference=w13265) -> ("Value"=w13263:T6)  [unwired: 1 in, 2 out]
          n5077 = for {
            N: 8 -> [_]
            tunnel: w13263 -> [w13275]
            shift-right: [w13277] -> w13269
            shift-left: dbl[] [] -> [w13273]
            i -> [w13276]
            n5078 = case shown="1" w13276 {
              tunnel: w13275 -> [w13278 w13289 w13300 w13312 w13322 w13333 w13345 w13356]
              tunnel: [w13279 w13290 w13301 w13313 w13324 w13335 w13347 w13357] -> w13274
              frame 0, Default {
                # "最大允许单体电压"
                n5079 = disable-structure shown="启用" {
                  disable-tunnel: [w13285 w13288] -> w13281
                  disable-tunnel: [w13284 w13288] -> w13280
                  disable-tunnel: w13278 -> [w13283 _]
                  frame Disabled {
                    n5080 = Unbundle By Name(w13283) -> ("最大允许单体电压"=w13282:dbl)
                    n5081 = call "输入分辨率计算-EV05.vi"("1字节?"=FALSE, "数值"=w13282, "分辨率"=0.001) -> ("低字节"=w13284:dbl, "高字节1"=w13285:dbl)  [unwired: 2 in, 5 out]
                  }
                  frame Enabled {
                    w13288 = 255 ("高字节1")
                  }
                }
                n5082 = Build Array(w13281, w13280) -> (w13279:i32[])
              }
              frame 1 {
                # "最大允许总电压"
                n5083 = disable-structure shown="启用" {
                  disable-tunnel: [w13296 w13299] -> w13292
                  disable-tunnel: [w13295 w13299] -> w13291
                  disable-tunnel: w13289 -> [w13294 _]
                  frame Enabled {
                    n5084 = Unbundle By Name(w13294) -> ("最大允许总电压"=w13293:dbl)
                    n5085 = call "输入分辨率计算-EV05.vi"("1字节?"=FALSE, "数值"=w13293, "分辨率"=0.1) -> ("低字节"=w13295:dbl, "高字节1"=w13296:dbl)  [unwired: 2 in, 5 out]
                  }
                  frame Disabled {
                    w13299 = 255 ("高字节1")
                  }
                }
                n5086 = Build Array(w13292, w13291) -> (w13290:dbl[])
              }
              frame 2 {
                # "最大允许充电电流"
                n5087 = disable-structure shown="启用" {
                  disable-tunnel: [w13308 w13311] -> w13303
                  disable-tunnel: [w13307 w13311] -> w13302
                  disable-tunnel: w13300 -> [w13305 _]
                  frame Disabled {
                    n5088 = Unbundle By Name(w13305) -> ("最大允许充电电流"=w13304:dbl)
                    n5089 = call "输入分辨率计算-EV05.vi"("1字节?"=FALSE, "数值"=w13304, "偏移量"=-3000.0, "分辨率"=0.1) -> ("低字节"=w13307:dbl, "高字节1"=w13308:dbl)  [unwired: 1 in, 5 out]
                  }
                  frame Enabled {
                    w13311 = 255 ("高字节1")
                  }
                }
                n5090 = Build Array(w13303, w13302) -> (w13301:i32[])
              }
              frame 3 {
                # "最小允许充电温度"
                n5091 = disable-structure shown="启用" {
                  disable-tunnel: [w13318 255 ("高字节1")] -> w13314
                  disable-tunnel: w13312 -> [w13316 _]
                  frame Disabled {
                    n5092 = Unbundle By Name(w13316) -> ("最小允许温度"=w13315:dbl)
                    n5093 = call "输入分辨率计算-EV05.vi"("1字节?"=TRUE, "数值"=w13315, "偏移量"=-40.0, "分辨率"=1.0) -> ("高字节1"=w13318:dbl)  [unwired: 1 in, 6 out]
                  }
                  frame Enabled {
                  }
                }
                n5094 = Build Array(w13314) -> (w13313:i32[])
              }
              frame 4 {
                # "最小充电电流"
                n5095 = disable-structure shown="启用" {
                  disable-tunnel: [w13329 w13332] -> w13325
                  disable-tunnel: [w13328 w13332] -> w13323
                  disable-tunnel: w13322 -> [w13327 _]
                  frame Disabled {
                    n5096 = Unbundle By Name(w13327) -> ("最小充电电流"=w13326:dbl)
                    n5097 = call "输入分辨率计算-EV05.vi"("1字节?"=FALSE, "数值"=w13326, "分辨率"=0.1) -> ("低字节"=w13328:dbl, "高字节1"=w13329:dbl)  [unwired: 2 in, 5 out]
                  }
                  frame Enabled {
                    w13332 = 255 ("高字节1")
                  }
                }
                n5098 = Build Array(w13325, w13323) -> (w13324:i32[])
              }
              frame 5 {
                # "电流步长"
                n5099 = disable-structure shown="启用" {
                  disable-tunnel: [w13341 w13344] -> w13336
                  disable-tunnel: [w13339 w13344] -> w13334
                  disable-tunnel: w13333 -> [w13338 _]
                  frame Disabled {
                    n5100 = Unbundle By Name(w13338) -> ("电流步长"=w13337:dbl)
                    n5101 = call "输入分辨率计算-EV05.vi"("1字节?"=FALSE, "数值"=w13337, "偏移量"=0.0, "分辨率"=1.0) -> ("低字节"=w13339:dbl, "高字节1"=w13341:dbl)  [unwired: 1 in, 5 out]
                  }
                  frame Enabled {
                    w13344 = 255 ("高字节1")
                  }
                }
                n5102 = Build Array(w13336, w13334) -> (w13335:i32[])
              }
              frame 6 {
                # "最小允许单体电压"
                n5103 = disable-structure shown="启用" {
                  disable-tunnel: [w13352 w13355] -> w13348
                  disable-tunnel: [w13351 w13355] -> w13346
                  disable-tunnel: w13345 -> [w13350 _]
                  frame Disabled {
                    n5104 = Unbundle By Name(w13350) -> ("最小允许单体电压"=w13349:dbl)
                    n5105 = call "输入分辨率计算-EV05.vi"("1字节?"=FALSE, "数值"=w13349, "分辨率"=0.001) -> ("低字节"=w13351:dbl, "高字节1"=w13352:dbl)  [unwired: 2 in, 5 out]
                  }
                  frame Enabled {
                    w13355 = 255 ("高字节1")
                  }
                }
                n5106 = Build Array(w13348, w13346) -> (w13347:i32[])
              }
              frame 7 {
                # "最大允许充电温度"
                n5107 = disable-structure shown="启用" {
                  disable-tunnel: [w13362 255 ("高字节1")] -> w13358
                  disable-tunnel: w13356 -> [w13360 _]
                  frame Disabled {
                    n5108 = Unbundle By Name(w13360) -> ("最大允许充电温度"=w13359:dbl)
                    n5109 = call "输入分辨率计算-EV05.vi"("1字节?"=TRUE, "数值"=w13359, "偏移量"=-40.0, "分辨率"=1.0) -> ("高字节1"=w13362:dbl)  [unwired: 1 in, 6 out]
                  }
                  frame Enabled {
                  }
                }
                n5110 = Build Array(w13358) -> (w13357:i32[])
              }
            }
            n5111 = Insert Into Array(array=w13273, new element=w13274) -> (w13277:dbl[])  [unwired: 1 in]
          }
          n5112 = Build Array(w13269) -> (w13271:dbl[][])
        }
        frame "最大允许充电电流" {
          n5113 = Unbundle By Name(w13369) -> ("充电控制参数"=w13370:refnum<vi>)
          n5114 = property class="Clust (严格)"(reference=w13370) -> ("Value"=w13368:T6)  [unwired: 1 in, 2 out]
          n5115 = for {
            N: 8 -> [_]
            tunnel: w13368 -> [w13380]
            shift-right: [w13382] -> w13374
            shift-left: dbl[] [] -> [w13378]
            i -> [w13381]
            n5116 = case shown="2" w13381 {
              tunnel: w13380 -> [w13383 w13394 w13405 w13417 w13427 w13438 w13450 w13461]
